vi "Waveform array sizing.vi"(8 "waveforms in":T1=array6x12000[72000 elements] format="%.2f", 10 "repeat period (ticks)":i32, 11 "number of channels":i32) -> (0 "waveforms out":T1 format="%.2f", 2 "last value":dbl[](array[numeric]) format="%.2f")   [LabVIEW 2010]
uses:
  wavecluster.ctl
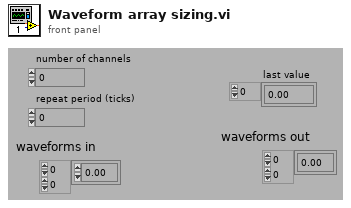
[diagram p1: front panel]
types:
  T1 = typedef "wavecluster.ctl" = sgl[][]
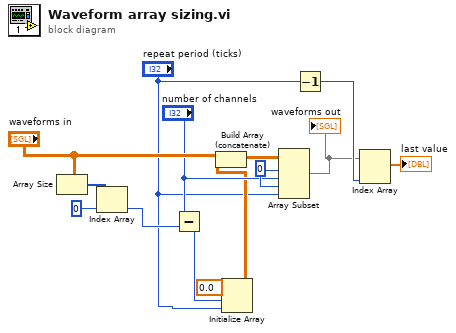
[diagram p0: block diagram]
diagram:
  w12 = 0 ("Array Index")
  n1 = Array Size(array="waveforms in") -> (size(s)=w11:i32[])
  n2 = Index Array(array=w11, index=0 ("Index")) -> (element=w7:i32)
  n3 = Subtract(x="number of channels", y=w7) -> (x-y=w6:i32)
  n4 = Initialize Array(0.0, w6, "repeat period (ticks)") -> (w2:dbl[][])
  n5 = Build Array (concatenate)("waveforms in", w2) -> (w9:dbl[][])
  n6 = Array Subset(array=w9, index (row)=w12, length (row)="number of channels", index (col)=w12, length (col)="repeat period (ticks)") -> (w4:dbl[][])
  "waveforms out" <- w4
  n7 = Decrement(x="repeat period (ticks)") -> (x-1=w13:i32)
  n8 = Index Array(array=w4, index (col)=w13) -> (element=→"last value":dbl[])  [unwired: 1 in]
